vi "Read SensorData Changed Event.vi"(8 "error in (no error)":errorcluster, 11 "SensorView in":refnum<class "SensorView.lvclass">) -> (0 "error out":errorcluster, 2 "SensorData Changed Event":refnum<user-event>, 3 "SensorView out":refnum<class "SensorView.lvclass">)   [LabVIEW 2012, in "Sensor Definition.lvlib" / "SensorView.lvclass"]
uses:
  SensorView.lvclass
  SensorData.lvclass
  SensorView.lvclass/SensorView.ctl
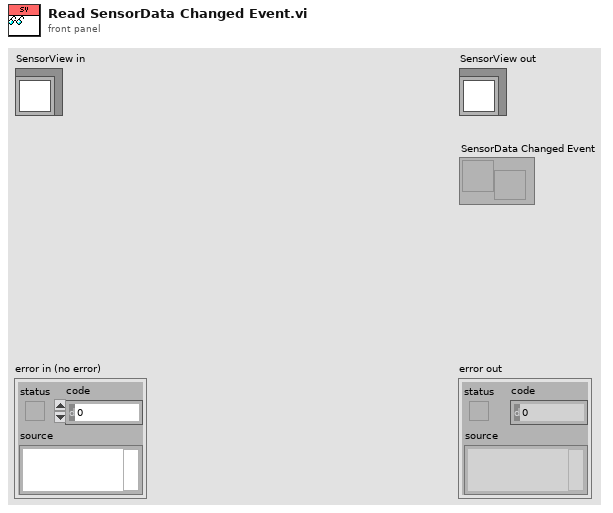
[diagram p1: front panel]
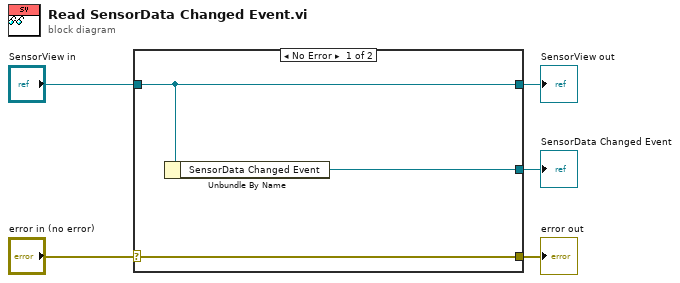
[diagram p0: block diagram]
diagram:
  n1 = case shown="No Error" "error in (no error)" {
    selector: "error in (no error)" -> [w8 w9]
    tunnel: [w8 w9] -> w4
    tunnel: [w7 w10] -> w2
    tunnel: "SensorView in" -> [w7 w10]
    tunnel: [w6 _] -> w1
    frame No Error {
      n2 = Unbundle By Name(w7) -> ("SensorData Changed Event"=w6:refnum<user-event>)
    }
    frame Error {
    }
  }
  "error out" <- w4
  "SensorView out" <- w2
  "SensorData Changed Event" <- w1
